vi "1.1 Poprawione.vi"(10 "n":u32) -> (2 "fib(n)":i32)   [LabVIEW 2013]
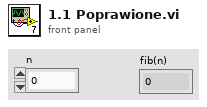
[diagram p1: front panel]
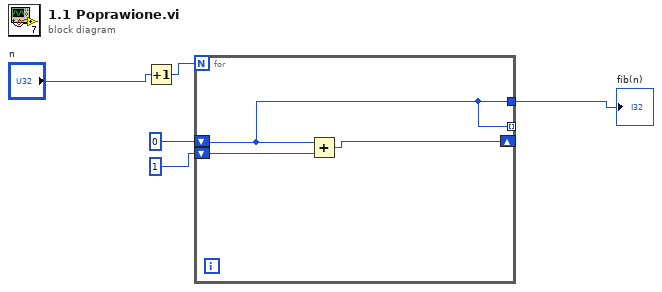
[diagram p0: block diagram]
diagram:
  n1 = Increment(x="n") -> (x+1=w5:u32)
  n2 = for {
    N: w5 -> [_]
    shift-right: [w7] -> _
    shift-left: 0 ("fib(n) 2") -> [w6]
    shift-left: 1 ("fib(n) 2") -> [w8]
    tunnel: [w6] -> w1
    tunnel: [w6] -> _ mode=indexing
    n3 = Add(x=w6, y=w8) -> (x+y=w7:i32)
  }
  "fib(n)" <- w1
